vi "GlobValue.vi"() -> ()   [LabVIEW 2013]
uses:
  Ctl/IOConfig.ctl
  Ctl/Setup.ctl
panel:
  in  "CCID":string[](array[string])
  in  "OtherCOM":refnum<visa-resource-name>
  in  "SlotQCCOM":refnum<visa-resource-name>
  in  "IOCOM":refnum<visa-resource-name>
  in  "SlotCOM":refnum<visa-resource-name>
  in  "PowerCOM":refnum<visa-resource-name>
  in  "SlotUSBCOM":refnum<visa-resource-name>
  in  "ConfigOut":T1={"TestedNum"=10, "PassedNum"=5, "FailedNum"=5, "Slot1TestedNum"=10, "Slot2TestedNum"=10, "Slot3TestedNum"=10, "Slot4TestedNum"=10, "GuiVer"="1.0", "LimitFileVer"="1.0", "Login Name"="", "Password"="", "SN_Head"="0", "SN_Length"=1, "AbortOnFail"=FALSE, "DataBaseEnable?"=FALSE, "FixtureID"="", "ShowSkipStep?"=FALSE}
  in  "通信协议":string[][](array[string])
  in  "测试项目":string[][](table)
  out "debug":bool
  out "Instruments":T2(array[cluster])
  in  "MainViPath":path
  in  "IOConfig":T3
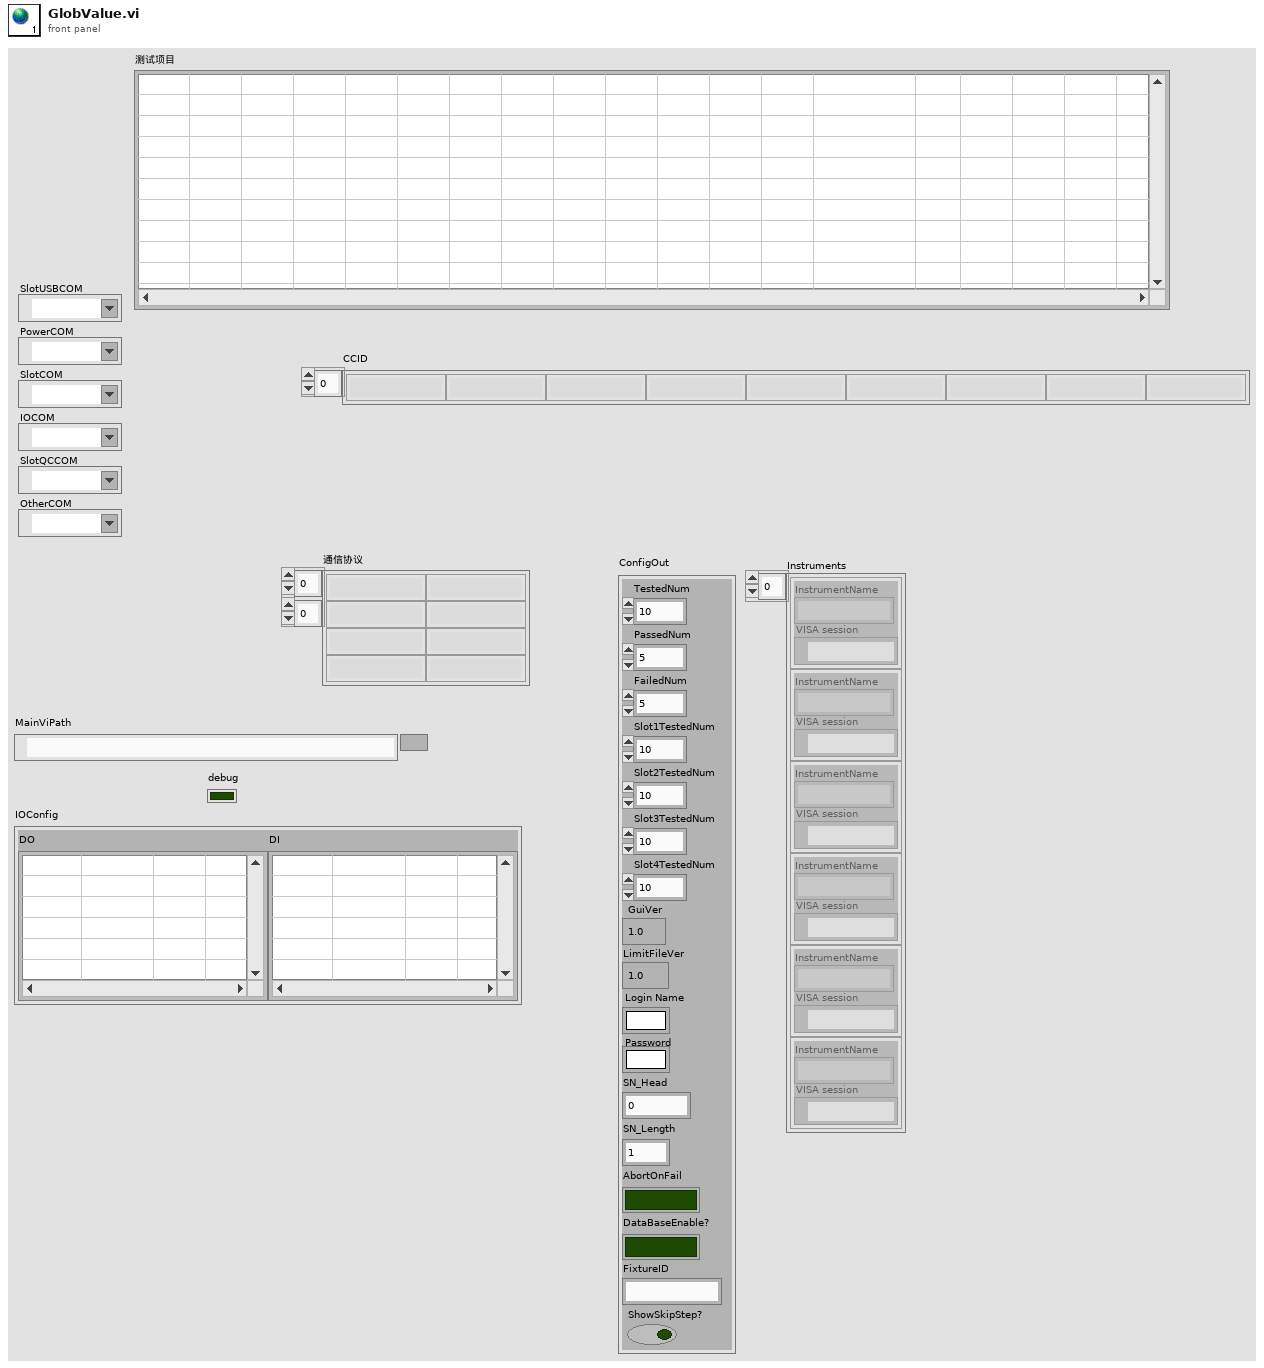
[diagram p1: front panel]
types:
  T1 = typedef "Setup.ctl" = cluster{"TestedNum":u32, "PassedNum":u32, "FailedNum":u32, "Slot1TestedNum":u32, "Slot2TestedNum":u32, "Slot3TestedNum":u32, "Slot4TestedNum":u32, "GuiVer":string, "LimitFileVer":string, "Login Name":string, "Password":string, "SN_Head":string, "SN_Length":i32, "AbortOnFail":bool, "DataBaseEnable?":bool, "FixtureID":string, "ShowSkipStep?":bool}
  T2 = cluster{"InstrumentName":string, "VISA session":refnum<visa-resource-name>}[]
  T3 = typedef "IOConfig.ctl" = cluster{"DO":string[][], "DI":string[][]}
diagram:
